vi "Kinect MAIN.vi"() -> ()   [LabVIEW 2014]
uses:
  <vilib>/University of Leeds/Kinesthesia Toolkit for Microsoft Kinect/_Polymorphic Configure/Event-Skeleton.vi
  <vilib>/University of Leeds/Kinesthesia Toolkit for Microsoft Kinect/_Polymorphic Read/Read-Skeleton.vi
  Kinect Global.vi
  <vilib>/University of Leeds/Kinesthesia Toolkit for Microsoft Kinect/_Polymorphic Close/Close-Skeleton.vi
panel:
  out "error out":errorcluster
  out "Loop time":u32=50
  out "3D Picture":refnum<vi>(3d-picture)
  in  "stop":bool
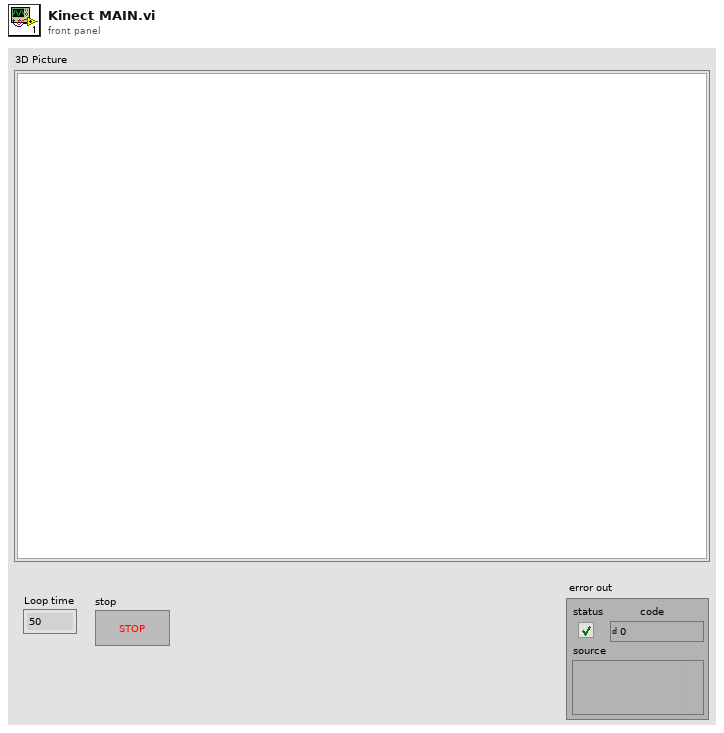
[diagram p1: front panel]
types:
  T1 = cluster{cluster{"reference out":refnum<k24>, "KinectSensors":refnum<k24>}, "get_Item":refnum<k24>}
  T2 = cluster{"Scene":refnum<vi>, "Joints":refnum<vi>[], "Bones":refnum<vi>[]}
  T3 = cluster{"reference out":refnum<k24>, "KinectSensors":refnum<k24>, "SkeletonStream":refnum<k24>, refnum<k24>[], "get_Item":refnum<k24>}
  T4 = typedef "Control cluster.ctl" = cluster{"Roll":sgl, "Pitch":sgl, "Vertical Speed":sgl, "Yaw Speed":sgl}
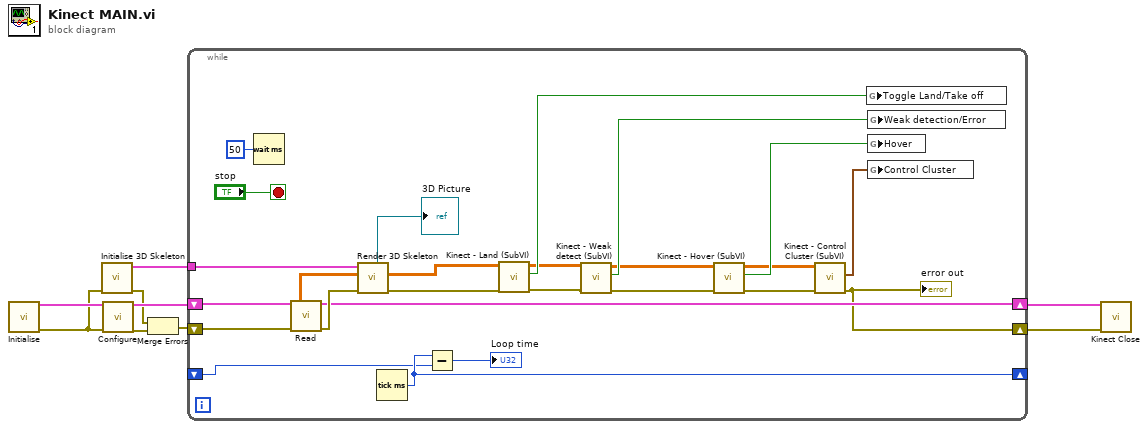
[diagram p0: block diagram]
diagram:
  n1 = call <vilib>:"Initialise.vi"() -> ("Kinect References out"=w9:T1, "error out"=w5:errorcluster)  [unwired: 14 in]
  n2 = call <vilib>:"Initialise 3D Skeleton.vi"("error in (no error)"=w5) -> ("error out"=w1:errorcluster, "Scene & Skeleton Refs"=w4:T2)  [unwired: 9 in]
  n3 = call-poly <vilib>:"Configure.vi"("Kinect References in"=w9, "error in"=w5) -> ("Kinect References out"=w8:T3, "error out"=w2:errorcluster)  [unwired: 12 in]
  n4 = Merge Errors(w1, w2) -> (w3:errorcluster)
  n5 = while {
    shift-right: [w13] -> w7
    shift-left: w8 -> [w18]
    shift-right: [w12] -> w6
    shift-left: w3 -> [w14]
    shift-right: [w34] -> _
    shift-left: _ -> [w33]
    tunnel: w4 -> [w17]
    stop <- "stop" stop-if-true
    n6 = Wait (ms)(milliseconds to wait=u32 50) -> ()  [unwired: 1 out]
    n7 = call-poly <vilib>:"Read.vi"("Kinect References in"=w18, "error in (no error)"=w14) -> ("Primary Skeleton Array"=w11:dbl[][], "Kinect References out"=w13:T3, "error out"=w15:errorcluster)  [unwired: 10 in, 1 out]
    n8 = call <vilib>:"Render 3D Skeleton.vi"("error in (no error)"=w15, "Array of Joint Positions"=w11, "Scene & Skeleton Refs In"=w17) -> ("error out"=w16:errorcluster, "Array of Joint Positions Out"=w26:dbl[][], "Scene Out"=→"3D Picture":refnum<vi>)  [unwired: 5 in, 1 out]
    n9 = Tick Count (ms)() -> (millisecond timer value=w34:u32)
    n10 = Subtract(x=w34, y=w33) -> (x-y=→"Loop time":u32)
    n11 = call "Kinect - Land (SubVI).vi"("error in (no error)"=w16, "Array of Joint Positions Out"=w26) -> ("error out"=w28:errorcluster, "Boolean"=w29:bool, "Array of Joint Positions Out 2"=w27:dbl[][])  [unwired: 6 in, 1 out]
    n12 = call "Kinect - Weak detect (SubVI).vi"("error in (no error)"=w28, "Array of Joint Positions In"=w27) -> ("error out"=w24:errorcluster, "Boolean"=w25:bool, "Array of Joint Positions Out"=w23:dbl[][])  [unwired: 6 in]
    n13 = call "Kinect - Hover (SubVI).vi"("error in (no error)"=w24, "Array of Joint Positions Out in"=w23) -> ("error out"=w21:errorcluster, "Boolean"=w22:bool, "Array of Joint Positions Out out"=w20:dbl[][])  [unwired: 7 in]
    n14 = call "Kinect - Control Cluster (SubVI).vi"("error in (no error)"=w21, "Array of Joint Positions in"=w20) -> ("error out"=w12:errorcluster, "Control Cluster out"=w19:T4)  [unwired: 6 in, 1 out]
    "error out" <- w12
    n15 = global write "Kinect Global.vi" "Toggle Land/Take off"(w29) -> ()
    n16 = global write "Kinect Global.vi" "Weak detection/Error"(w25) -> ()
    n17 = global write "Kinect Global.vi" "Hover"(w22) -> ()
    n18 = global write "Kinect Global.vi" "Control Cluster"(w19) -> ()
  }
  n19 = call-poly <vilib>:"Kinect Close.vi"("Kinect References in"=w7, "error in"=w6) -> ()  [unwired: 13 in, 1 out]
